vi "WPI_ReserveFilterResource.vi"(8 "error in (no error)":errorcluster, 9 "Release Filter":bool, 10 "Filter Period":u32, 11 "DigitalInputDevRef":T1={"DevStatus"={"status"=FALSE, "code"=0, "source"=""}, "DIO Channel"=enum."DIO 1"}) -> (0 "error out":errorcluster, 2 "Filter Index":u8, 3 "DigitalInputDevRef":T1={"DevStatus"={"status"=FALSE, "code"=0, "source"=""}, "DIO Channel"=enum."DIO 1"})   [LabVIEW 2017]
uses:
  <vilib>/Rock Robotics/WPI/DigitalInput/WPI_DigitalInputDevRef.ctl
  <vilib>/Rock Robotics/SystemInterfaces/DIO/FPGA_DIOChannel.ctl
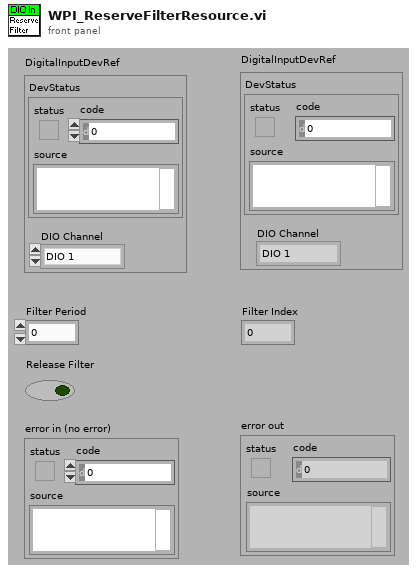
[diagram p1: front panel]
types:
  T1 = typedef "WPI_DigitalInputDevRef.ctl" = cluster{"DevStatus":errorcluster, "DIO Channel":T2}
  T2 = typedef "FPGA_DIOChannel.ctl" = enum8{"DIO 0", "DIO 1", "DIO 2", "DIO 3", "DIO 4", "DIO 5", "DIO 6", "DIO 7", "DIO 8", "DIO 9", "DIO MXP 0", "DIO MXP 1", "DIO MXP 2", "DIO MXP 3", "DIO MXP 4", "DIO MXP 5", "DIO MXP 6", "DIO MXP 7", "DIO MXP 8", "DIO MXP 9", "DIO MXP 10", "DIO MXP 11", "DIO MXP 12", "DIO MXP 13", "DIO MXP 14", "DIO MXP 15", "SPI Port CS1", "SPI Port CS2", "SPI Port CS3", "SPI Port MISO", "SPI Port MOSI", "Invalid"}
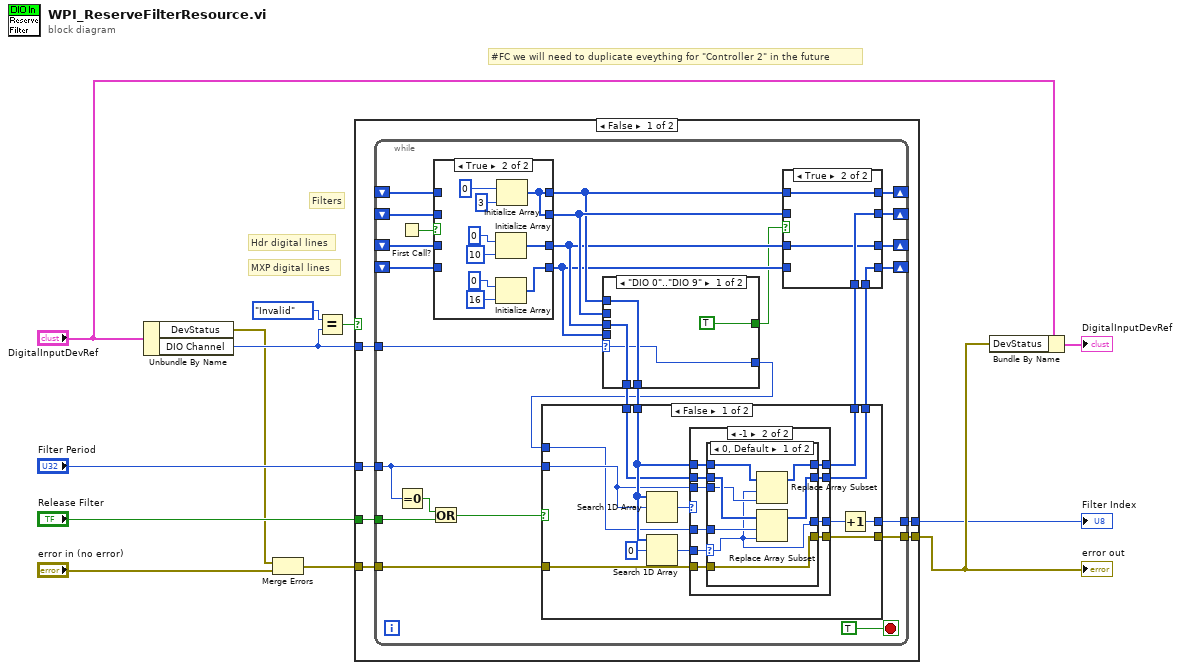
[diagram p0: block diagram]
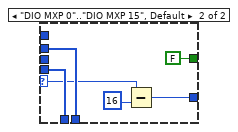
[diagram p3: hidden frame]
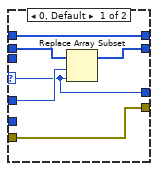
[diagram p5: hidden frame]
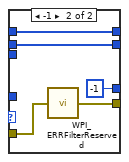
[diagram p6: hidden frame]
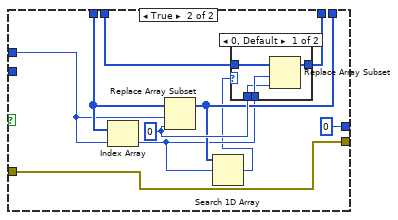
[diagram p7: hidden frame]
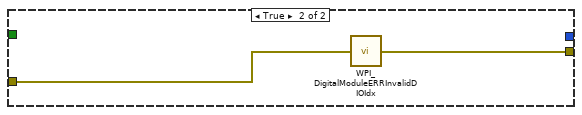
[diagram p9: hidden frame]
diagram:
  # "MXP digital lines"
  # "Hdr digital lines"
  # "Filters"
  # "#FC we will need to duplicate eveything for \"Controller 2\" in the future"
  n1 = Unbundle By Name("DigitalInputDevRef") -> ("DevStatus"=w2:errorcluster, "DIO Channel"=w11:T2)
  n2 = Merge Errors(w2, "error in (no error)") -> (w1:errorcluster)
  n3 = Equal?(x=FPGA_DIOChannel."Invalid" ("DIO Channel"), y=w11) -> (x = y?=w4:bool)
  n4 = case shown="False" w4 {
    tunnel: "Release Filter" -> [w18 _]
    tunnel: "Filter Period" -> [w17 _]
    tunnel: [w16 w136] -> w8
    tunnel: w11 -> [w15 _]
    tunnel: [w14 _] -> w6
    tunnel: w1 -> [w13 w135]
    frame False {
      n5 = while {
        shift-right: [w39] -> _
        shift-left: _ -> [w43]
        tunnel: w18 -> [w45]
        shift-right: [w38] -> _
        shift-left: _ -> [w42]
        tunnel: w15 -> [w21]
        tunnel: w17 -> [w27]
        shift-right: [w32] -> _
        shift-left: _ -> [w35]
        shift-right: [w33] -> _
        shift-left: _ -> [w34]
        tunnel: [w24] -> w16
        tunnel: [w23] -> w14
        tunnel: w13 -> [w22]
        stop <- TRUE stop-if-true
        n6 = First Call?() -> (First Call?: T/F=w44:bool)
        n7 = Equal To 0?(x=w27) -> (x = 0?=w25:bool)
        n8 = Or(x=w25, y=w45) -> (x .or. y?=w26:bool)
        n9 = case shown="True" w44 {
          tunnel: w43 -> [w68 _]
          tunnel: [w68 w76] -> w40
          tunnel: w42 -> [w67 _]
          tunnel: [w67 w76] -> w41
          tunnel: w35 -> [w66 _]
          tunnel: w34 -> [w65 _]
          tunnel: [w66 w70] -> w31
          tunnel: [w65 w69] -> w30
          frame False {
          }
          frame True {
            n10 = Initialize Array(u32 0, 10 ("dimension size")) -> (w70:u32[])
            n11 = Initialize Array(u32 0, 16 ("dimension size")) -> (w69:u32[])
            n12 = Initialize Array(u32 0, 3 ("dimension size")) -> (w76:u32[])
          }
        }
        n13 = case shown="\"DIO 0\"..\"DIO 9\"" w21 {
          selector: w21 -> [w55 w61]
          tunnel: w40 -> [w58 _]
          tunnel: w41 -> [_ w64]
          tunnel: [w58 w64] -> w36
          tunnel: w31 -> [w57 _]
          tunnel: w30 -> [_ w63]
          tunnel: [w57 w63] -> w29
          tunnel: [TRUE FALSE] -> w20
          tunnel: [w55 w60] -> w19
          frame "DIO 0".."DIO 9" {
          }
          frame "DIO MXP 0".."DIO MXP 15", Default {
            n14 = Subtract(x=w61, y=u8 16) -> (x-y=w60:u8)
          }
        }
        n15 = case shown="False" w26 {
          tunnel: [w86 w126] -> w37
          tunnel: w36 -> [w85 w127]
          tunnel: w29 -> [w83 w129]
          tunnel: [w84 w124] -> w28
          tunnel: w19 -> [w81 w128]
          tunnel: w27 -> [w82 _]
          tunnel: [w87 w120] -> w24
          tunnel: [w79 0 ("index of element")] -> w23
          tunnel: w22 -> [w78 w120]
          frame False {
            n16 = Search 1D Array(1D array=w85, element=w82) -> (index of element=w89:i32)  [unwired: 1 out]
            n17 = Search 1D Array(1D array=w85, element=u32 0) -> (index of element=w88:i32)  [unwired: 1 out]
            n18 = case shown="-1" w89 {
              selector: w89 -> [w92 _]
              tunnel: w88 -> [_ w106]
              tunnel: [w91 w105] -> w87
              tunnel: [w96 w104] -> w86
              tunnel: w85 -> [w96 w103]
              tunnel: [w94 w102] -> w84
              tunnel: w83 -> [w95 w101]
              tunnel: w82 -> [_ w100]
              tunnel: w81 -> [w93 w99]
              tunnel: [w92 w98] -> w80
              tunnel: w78 -> [w91 w97]
              frame 0, Default {
                n19 = Replace Array Subset(array=w95, new element=w92, index=w93) -> (w94:u32[])
              }
              frame -1 {
                n20 = case shown="0, Default" w106 {
                  selector: w106 -> [w108 _]
                  tunnel: [w107 w119] -> w105
                  tunnel: [w111 w118] -> w104
                  tunnel: w103 -> [w112 w118]
                  tunnel: [w113 w117] -> w102
                  tunnel: w101 -> [w114 w117]
                  tunnel: w100 -> [w110 _]
                  tunnel: w99 -> [w109 _]
                  tunnel: [w108 -1 ("index of element")] -> w98
                  tunnel: w97 -> [w107 w115]
                  frame 0, Default {
                    n21 = Replace Array Subset(array=w112, new element=w110, index=w108) -> (w111:u32[])
                    n22 = Replace Array Subset(array=w114, new element=w108, index=w109) -> (w113:u32[])
                  }
                  frame -1 {
                    n23 = call <vilib>:"WPI_ERRFilterReserved.vi"("error in (no error)"=w115) -> ("error out"=w119:errorcluster)
                  }
                }
              }
            }
            n24 = Increment(x=w80) -> (x+1=w79:i32)
          }
          frame True {
            w125 = u32 0 ("new element/subarray")
            n25 = Index Array(array=w129, index=w128) -> (element=w123:u32)
            n26 = Replace Array Subset(array=w129, new element=w125, index=w128) -> (w124:u32[])
            n27 = Search 1D Array(1D array=w124, element=w123) -> (index of element=w122:i32)  [unwired: 1 out]
            n28 = case shown="0, Default" w122 {
              tunnel: w127 -> [w133 w134]
              tunnel: [w132 w134] -> w126
              tunnel: w123 -> [w131 _]
              tunnel: w125 -> [w130 _]
              frame 0, Default {
                n29 = Replace Array Subset(array=w133, new element=w130, index=w131) -> (w132:u32[])
              }
              frame -1 {
              }
            }
          }
        }
        n30 = case shown="True" w20 {
          tunnel: w41 -> [w50 _]
          tunnel: w40 -> [_ w54]
          tunnel: [w49 w54] -> w39
          tunnel: [w50 w53] -> w38
          tunnel: w37 -> [w49 w53]
          tunnel: w31 -> [_ w52]
          tunnel: [w48 w51] -> w33
          tunnel: w30 -> [w48 _]
          tunnel: [w47 w52] -> w32
          tunnel: w28 -> [w47 w51]
          frame False {
          }
          frame True {
          }
        }
      }
    }
    frame True {
      n31 = call <vilib>:"WPI_DigitalModuleERRInvalidDIOIdx.vi"("error in (no error)"=w135) -> ("error out"=w136:errorcluster)
    }
  }
  "Filter Index" <- w6
  "error out" <- w8
  n32 = Bundle By Name(cluster="DigitalInputDevRef", "DevStatus"=w8) -> (→"DigitalInputDevRef":T1)
